vi "Read Timeout.vi"(8 "error in (no error)":errorcluster, 11 "OnChange_Boolean in":refnum<class "OnChange_Boolean.lvclass">) -> (0 "error out":errorcluster, 2 "Timeout":bool, 3 "OnChange_Boolean out":refnum<class "OnChange_Boolean.lvclass">)   [LabVIEW 2021, in "OnChange_Boolean.lvclass"]
uses:
  OnChange_Boolean.lvclass
  OnChange_Boolean.lvclass/OnChange_Boolean.ctl
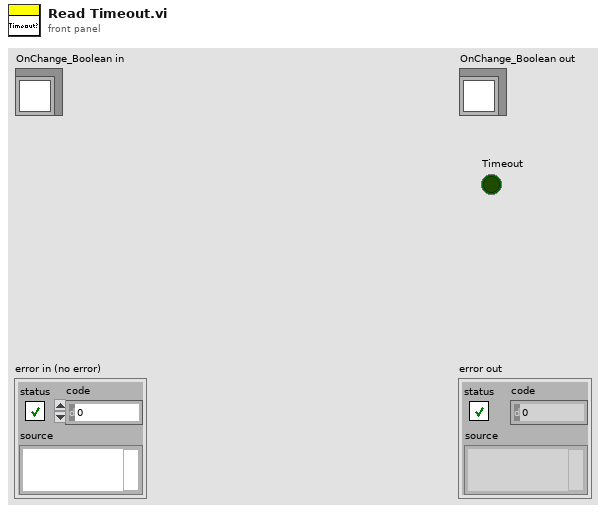
[diagram p1: front panel]
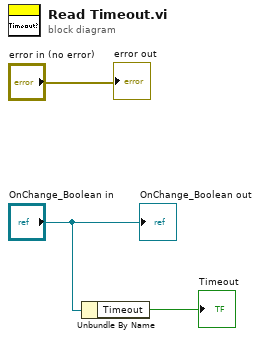
[diagram p0: block diagram]
diagram:
  n1 = Unbundle By Name("OnChange_Boolean in") -> ("Timeout"=→"Timeout":bool)
  "error out" <- "error in (no error)"
  "OnChange_Boolean out" <- "OnChange_Boolean in"
